vi "Read LVCluster by MoveBlock.vi"() -> ()   [LabVIEW 2012]
uses:
  demo dll.dll
panel:
  out "Destination":cluster{"U8":u8, "I32":i32, "DBL":dbl}
  in  "Pack1Cluster":cluster{"U8":u8, "I32":i32, "DBL":dbl}
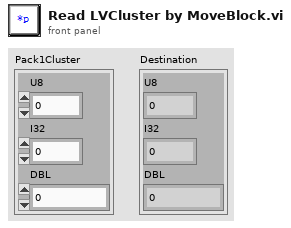
[diagram p1: front panel]
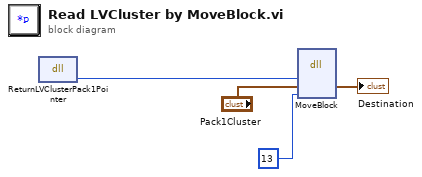
[diagram p0: block diagram]
diagram:
  n1 = dll-call lib="PTH1+abs EBOOK\t功能块DLLdemo dll.dll" fn="ReturnLVClusterPack1Pointer"() -> ("返回类型"=w4:u64)  [unwired: 3 in, 2 out]
  n2 = dll-call lib="LabVIEW" fn="MoveBlock"("Address (Pointer)"=w4, "Destination"="Pack1Cluster", "Size"=13) -> ("Destination"=→"Destination":cluster{"U8":u8, "I32":i32, "DBL":dbl})  [unwired: 6 in, 2 out]
